vi "Create Session.vi"(5 "advanced-http-client in":refnum<class "advanced-http-client.lvclass">, 6 "verify server (true)":bool, 7 "cookie file":path, 8 "error in (no error)":errorcluster, 9 "password":string, 10 "username":string) -> (0 "error out":errorcluster, 3 "advanced-http-client out":refnum<class "advanced-http-client.lvclass">)   [LabVIEW 2020, in "advanced-http-client.lvclass"]
uses:
  advanced-http-client.lvclass
  advanced-http-client.lvclass/advanced-http-client.ctl
  <vilib>/NI/Advanced HTTP Client/Session.lvclass
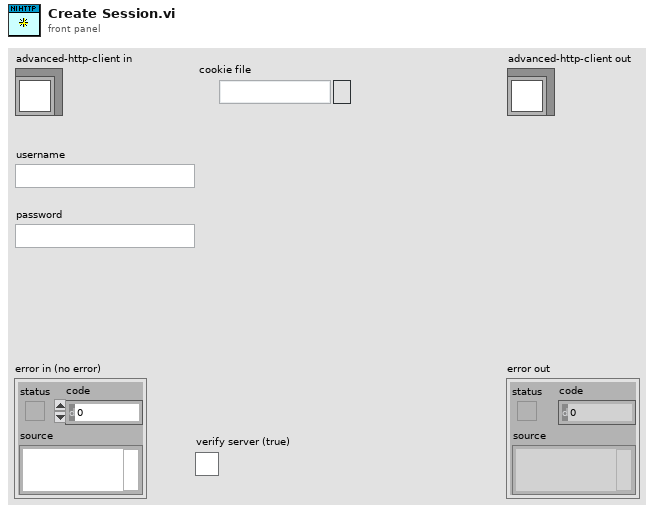
[diagram p1: front panel]
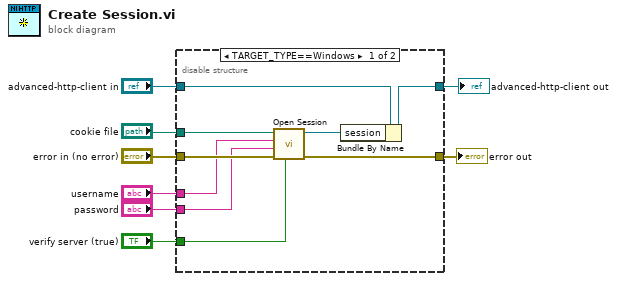
[diagram p0: block diagram]
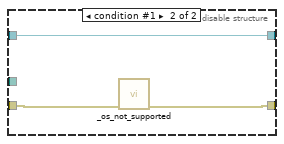
[diagram p2: hidden frame]
diagram:
  n1 = disable-structure shown="TARGET_TYPE==Windows" {
    disable-tunnel: "advanced-http-client in" -> [w17 w20]
    disable-tunnel: [w16 w20] -> w7
    disable-tunnel: "cookie file" -> [w15 _]
    disable-tunnel: [w13 w19] -> w5
    disable-tunnel: "verify server (true)" -> [w12 _]
    disable-tunnel: "error in (no error)" -> [w11 w18]
    disable-tunnel: "password" -> [w10 _]
    disable-tunnel: "username" -> [w9 _]
    frame condition #0 (active) {
      n2 = call <vilib>:"Open Session.vi"("verify server (T)"=w12, "error in"=w11, "password"=w10, "username"=w9, "cookie file"=w15) -> ("error out"=w13:errorcluster, "session"=w14:refnum<class "Session.lvclass">)  [unwired: 5 in]
      n3 = Bundle By Name(cluster=w17, "session"=w14) -> (w16:refnum<class "advanced-http-client.lvclass">)
    }
    frame condition #1 {
      n4 = call "_os_not_supported.vi"("error in (no error)"=w18) -> ("error out"=w19:errorcluster)  [unwired: 9 in, 1 out]
    }
  }
  "error out" <- w5
  "advanced-http-client out" <- w7
